vi "StartMeasurement.vi"(6 "First Measurement?":bool, 7 "MH_UIThread_Data":T1 {"Acquisitions" min=0 max=100000000 step=1; "T2 Coincidence Cluster"."Stdev" format="%0.2f"; "T2 Coincidence Cluster"."Mean" format="%0.2f"; "Mode" items=["HIST"=0, "T2"=2, "T3"=3]; "SyncDeadTime" min=800 max=160000 step=1; "SyncEdge" items=["falling", "rising"]; "SyncDivider" items=["1", "2", "4", "8", "16"]; "SyncOffset" min=0 max=100000 step=1; "SyncLevel" min=0 max=800 step=1; "AcqTime" min=1 max=360000 step=1; "Binning" items=["1", "2", "4", "8", "16", "32", "64", "128", "256", "512", "1024", "2048", "4096", "8192", "16384", "32768", "65536", "131072", "262144", "524288", "1048576", "2097152", "4194304", "8388608", "16777216", "3355443225"]; "HistoOffset" min=0 max=500 step=1; "HistoLen" min=1024 max=65536 step=1024; "Channels"."DeadTime" min=800 max=160000 step=1; "Channels"."Edge" items=["falling", "rising"]; "Channels"."Offset" min=-100000 max=100000 step=10; "Channels"."Level" min=-1200 max=1200 step=1}, 8 "error in (no error)":errorcluster, 10 "VI reference":refnum<vi>, 11 "Multiharp Enqueuer":refnum<class "Message Enqueuer.lvclass">) -> (0 "error out":errorcluster, 3 "MH_UIThread_Data":T1 {"Acquisitions" min=0 max=100000000 step=1; "T2 Coincidence Cluster"."Stdev" format="%0.2f"; "T2 Coincidence Cluster"."Mean" format="%0.2f"; "Mode" items=["HIST"=0, "T2"=2, "T3"=3]; "SyncDeadTime" min=800 max=160000 step=1; "SyncEdge" items=["falling", "rising"]; "SyncDivider" items=["1", "2", "4", "8", "16"]; "SyncOffset" min=0 max=100000 step=1; "SyncLevel" min=0 max=800 step=1; "AcqTime" min=1 max=360000 step=1; "Binning" items=["1", "2", "4", "8", "16", "32", "64", "128", "256", "512", "1024", "2048", "4096", "8192", "16384", "32768", "65536", "131072", "262144", "524288", "1048576", "2097152", "4194304", "8388608", "16777216", "3355443225"]; "HistoOffset" min=0 max=500 step=1; "HistoLen" min=1024 max=65536 step=1024; "Channels"."DeadTime" min=800 max=160000 step=1; "Channels"."Edge" items=["falling", "rising"]; "Channels"."Offset" min=-100000 max=100000 step=10; "Channels"."Level" min=-1200 max=1200 step=1})   [LabVIEW 2023, in "SinglePhotonInterferenceUI.lvlib" / "SinglePhotonInterferenceUI.lvclass"]
uses:
  SinglePhotonInterferenceUI.lvclass
  ConcreteClasses/ConcreteInstrumentClasses/Multiharp/Multiharp/Multiharp Messages/StartMeasurement Msg/StartMeasurement Msg.lvclass
  ConcreteClasses/ConcreteInstrumentClasses/Multiharp/Multiharp/_lib/PQ/MultiHarp/MH_InitInfo.ctl
  typedefs/typedefs.lvlib
  ConcreteClasses/ConcreteInstrumentClasses/Multiharp/Multiharp/Types/MH_InputChannel.ctl
  ConcreteClasses/ConcreteInstrumentClasses/Multiharp/Multiharp/Types/MH_SetInpChanCmds.ctl
  ConcreteClasses/ConcreteInstrumentClasses/Multiharp/Multiharp/Types/MH_SetInpChanData.ctl
  ConcreteClasses/ConcreteInstrumentClasses/Multiharp/Multiharp/_lib/PQ/MultiHarp/MH_MeasMode.ctl
  ConcreteClasses/ConcreteInstrumentClasses/Multiharp/Multiharp/Types/MH_UIThread_Data_SPI.ctl
  <vilib>/ActorFramework/Message Enqueuer/Message Enqueuer.lvclass
panel:
  # "Sync"
  # "Histogram"
  # "Sync"
  # "Histogram"
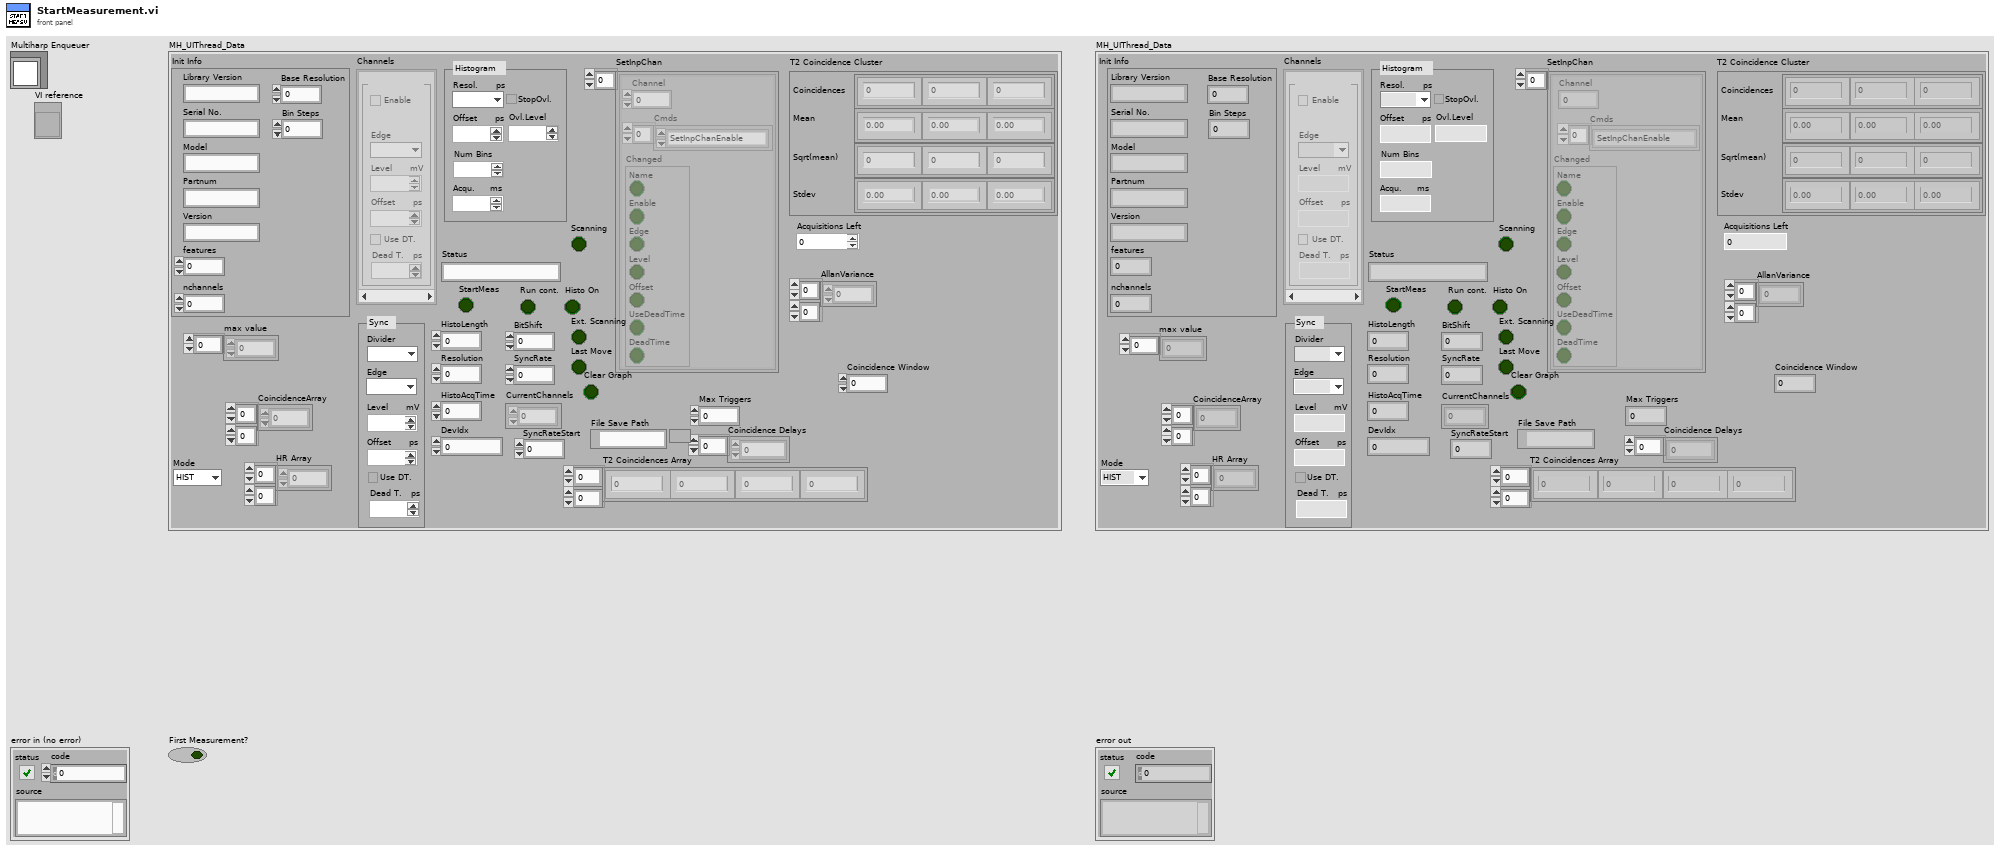
[diagram p1: front panel]
types:
  T1 = typedef "MH_UIThread_Data_SPI.ctl" = cluster{"Init Info":T2, "DevIdx":i32, "SyncDivider":i32, "SyncOffset":i32, "SyncLevel":i32, "Channels":T3[], "CurrentChannels":i32[], "AcqTime":i32, "Binning":i32, "HistoOffset":i32, "HistoLen":i32, "StopOvl.":bool, "OvlLevel":u32, "SyncEdge":i32, "StartMeas":bool, "HistoLength":i32, "Resolution":dbl, "Run cont.":bool, "Status":string, "SyncRate":i32, "BitShift":i32, "HistoAcqTime":dbl, "SyncRateStart":i32, "UseDeadTime":bool, "SyncDeadTime":i32, "SetInpChan":T4[], "max value":u32[], "CoincidenceArray":u32[][], "Histo On":bool, "Mode":T6, "Scanning":bool, "Last Move":bool, "Coincidence Window":dbl, "Max Triggers":i32, "Coincidence Delays":dbl[], "T2 Coincidences Array":i32[][], "Clear Graph":bool, "File Save Path":path, "T2 Coincidence Cluster":cluster{"Coincidences":u32[], "Mean":dbl[], "Sqrt(mean)":dbl[], "Stdev":dbl[]}, "Acquisitions":i32, "HR Array":sgl[][], "Ext. Scanning":bool, "AllanVariance":dbl[][]}
  T2 = typedef "typedefs.lvlib/MH_InitInfo.ctl" = cluster{"Library Version":string, "Serial No.":string, "Model":string, "Partnum":string, "Version":string, "features":i32, "nchannels":i32, "Base Resolution":dbl, "Bin Steps":i32}
  T3 = typedef "MH_InputChannel.ctl" = cluster{"Name":string, "Enable":bool, "Edge":i32, "Level":i32, "Offset":i32, "UseDeadTime":bool, "DeadTime":i32}
  T4 = typedef "MH_SetInpChanData.ctl" = cluster{"Channel":i32, "Cmds":T5[], "Changed":cluster{"Name":bool, "Enable":bool, "Edge":bool, "Level":bool, "Offset":bool, "UseDeadTime":bool, "DeadTime":bool}}
  T5 = typedef "MH_SetInpChanCmds.ctl" = enum16{"SetInpChanEnable", "SetInpChanOffset", "SetInpChanDeadTime", "SetInpChanTrg"}
  T6 = typedef "MH_MeasMode.ctl" = i32
  T7 = enum8{"Enabled", "Disabled", "Disabled and Grayed Out"}
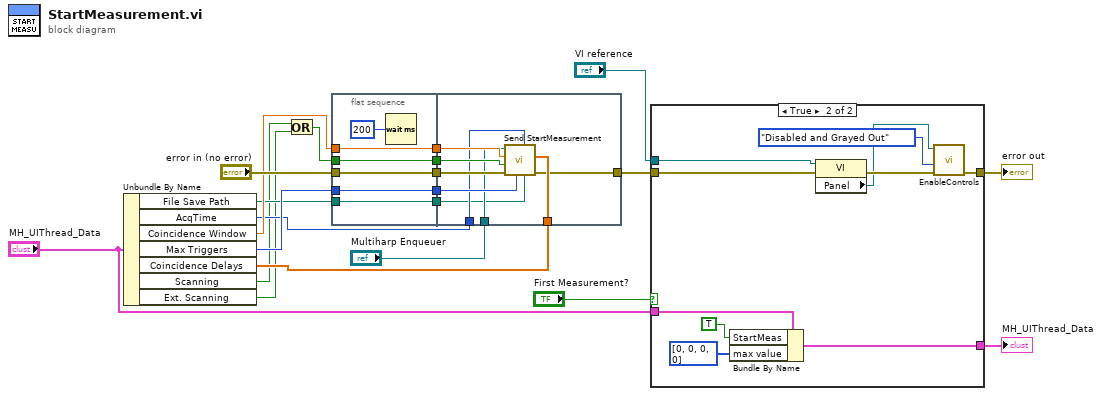
[diagram p0: block diagram]
diagram:
  n1 = Unbundle By Name("MH_UIThread_Data") -> ("File Save Path"=w12:path, "AcqTime"=w17:i32, "Coincidence Window"=w18:dbl, "Max Triggers"=w19:i32, "Coincidence Delays"=w21:dbl[], "Scanning"=w3:bool, "Ext. Scanning"=w2:bool)
  n2 = Or(x=w3, y=w2) -> (x .or. y?=w1:bool)
  n3 = flat-sequence {
    tunnel: w12 -> [w23]
    tunnel: w18 -> [w24]
    tunnel: w19 -> [w25]
    tunnel: w1 -> [w26]
    tunnel: "error in (no error)" -> [w27]
    tunnel: [w27] -> w8
    tunnel: [w26] -> w7
    tunnel: [w25] -> w6
    tunnel: [w24] -> w5
    tunnel: [w23] -> w4
    tunnel: w21 -> [w36]
    tunnel: w17 -> [w31]
    tunnel: "Multiharp Enqueuer" -> [w30]
    tunnel: [w28] -> w11
    tunnel: w8 -> [w35]
    tunnel: w7 -> [w34]
    tunnel: w6 -> [w33]
    tunnel: w5 -> [w32]
    tunnel: w4 -> [w29]
    frame #0 {
      n4 = Wait (ms)(milliseconds to wait=u32 200) -> ()  [unwired: 1 out]
    }
    frame #1 {
      n5 = call "Send StartMeasurement.vi"("Coincidence Delays"=w36, "Path"=w29, "tacq"=w31, "Max Triggers"=w33, "error in (no error)"=w35, "Scanning"=w34, "Coincidence Window"=w32, "Message Enqueuer"=w30) -> ("error out"=w28:errorcluster)  [unwired: 2 in, 1 out]
    }
  }
  n6 = case shown="True" "First Measurement?" {
    tunnel: [w37 w48] -> w16
    tunnel: "MH_UIThread_Data" -> [w37 w47]
    tunnel: w11 -> [w38 w41]
    tunnel: [w38 w40] -> w10
    tunnel: "VI reference" -> [_ w39]
    frame False {
    }
    frame True {
      n7 = Bundle By Name(cluster=w47, "StartMeas"=TRUE, "max value"=u32[] [0, 0, 0, 0]) -> (w48:T1)
      n8 = property class="VI"(reference=w39, error in=w41) -> (error out=w44:errorcluster, "Panel"=w43:refnum<vi>)  [unwired: 1 out]
      n9 = call "EnableControls.vi"("error in (no error)"=w44, "Disabled"=T7."Disabled and Grayed Out", "Panel in"=w43) -> ("error out"=w40:errorcluster)  [unwired: 8 in]
    }
  }
  "MH_UIThread_Data" <- w16
  "error out" <- w10
